vi "SimpleTest.vi"() -> ()   [LabVIEW 2020]
panel:
  out "error out":errorcluster
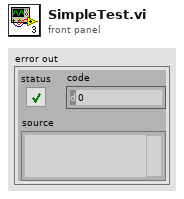
[diagram p1: front panel]
types:
  T1 = cluster{"IP Address":string, "Username":string, "password":string}
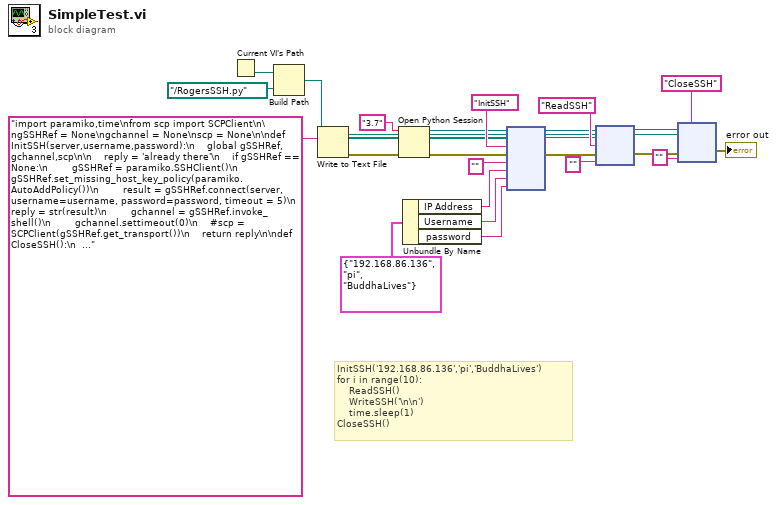
[diagram p0: block diagram]
diagram:
  # "InitSSH('192.168.86.136','pi','BuddhaLives')\nfor i in range(10):\n    ReadSSH()\n    WriteSSH('\\n\\n')\n    time.sleep(1)\nCloseSSH()"
  n1 = Current VI's Path() -> (path=w21:path)
  n2 = Build Path(base path=w21, name or relative path=path "../RogersSSH.py" ("base path")) -> (appended path=w3:path)
  n3 = Write to Text File(file (use dialog)=w3, text="import paramiko,time\nfrom scp import SCPClient\n\ngSSHRef = None\ngchannel = None\nscp = None\n\ndef InitSSH(server,username,password):\n    global gSSHRef, gchannel,scp\n\n    reply = 'already there'\n    if gSSHRef == None:\n        gSSHRef = paramiko.SSHClient()\n        gSSHRef.set_missing_host_key_policy(paramiko.AutoAddPolicy())\n        result = gSSHRef.connect(server, username=username, password=password, timeout = 5)\n        reply = str(result)\n        gchannel = gSSHRef.invoke_shell()\n        gchannel.settimeout(0)\n    #scp = SCPClient(gSSHRef.get_transport())\n    return reply\n\ndef CloseSSH():\n    if gchannel != None:\n        gchannel.close()\n    if gSSHRef != None:\n        gSSHRef.close()\n    if scp != None:\n        scp.close()\n    return('done')\n\ndef WriteSSH(string):\n    global gSSHRef, gchannel,scp\n    reply = 'no reference'\n    if gSSHRef != None:\n        reply = 'no file'\n        if gchannel != None:\n            size = gchannel.send(string.encode())\n            reply = str(size)\n    return reply\n\ndef ReadSSH():\n    global gSSHRef, gchannel,scp\n    reply = 'no reference'\n    if gSSHRef != None:\n        reply = 'no file'\n        if gchannel != None:\n            reply = ''\n            if gchannel.recv_ready():\n                reply = gchannel.recv(9999).decode()\n\n    return(reply)\n\ndef WriteWaitReadSSH(string,char,timeout=10000):\n     global gSSHRef, gchannel,scp\n     reply = ReadSSH()\n     WriteSSH(string)\n     n = int(timeout/10)\n     for i in range(n):\n         ans = ReadSSH()\n         reply = reply + ans\n         if ans.find(char) >= 0:\n             #print(ans)\n             return reply\n         time.sleep(0.01)\n     return reply\n\ndef scp_get(name):\n     try:\n          scp.get(name)\n          return 'get succeeded\\n'\n     except Exception as e:\n          return  'scp.get('+name+')\\n' +str(e)\n\ndef scp_put(source, dest):\n     try:\n          scp.put(source, dest)\n          return 'scp.put('+source+','+dest+')\\n' +'put succeeded\\n'\n     except Exception as e:\n          return str(e)\n\ndef scp_put_all(source, dest):\n     try:\n          scp.put(source, recursive = True, remote_path = dest)\n          return 'put succeeded\\n'\n     except Exception as e:\n          return str(e)\n" ("name or relative path")) -> (error out=w23:errorcluster)  [unwired: 2 in, 2 out]
  n4 = Open Python Session(python version="3.7" ("Python version"), 3:w23) -> (session out=w13:refnum<k35>, error out=w12:errorcluster)  [unwired: 1 in]
  n5 = Unbundle By Name(T1 {"IP Address"="192.168.86.136", "Username"="pi", "password"="BuddhaLives"} ("Raspberry Pi")) -> ("IP Address"=w16:string, "Username"=w15:string, "password"=w14:string)
  n6 = node(w13, w3, "InitSSH" ("function name"), w12, "" ("function name"), w16, w15, w14) -> (w8:refnum<k35>, w7:errorcluster)  [unwired: 4 in, 2 out]
  n7 = node(w8, w3, "ReadSSH" ("function name"), w7, "" ("replace string (\"\")")) -> (w4:refnum<k35>, w2:errorcluster)  [unwired: 1 in, 2 out]
  n8 = node(w4, w3, "CloseSSH" ("function name"), w2, "" ("function name")) -> (→"error out":errorcluster)  [unwired: 1 in, 3 out]
